vi "DataProcess.vi"(11 "Scan parameters":T1={"area/um"=36.9778, "range_x/v"=0.6347, "range_y/v"=0.7773, "interval/um"=0.1, "x_center/v"=3.35, "y_center/v"=5.55, "theta_1/de"=0.0, "theta_2/de"=60.0, "theta_3/de"=120.0}) -> (0 "ystart":dbl, 1 "xstart":dbl, 2 "ystep":dbl, 3 "xstep":dbl, 5 "NUM":i32)   [LabVIEW 2014]
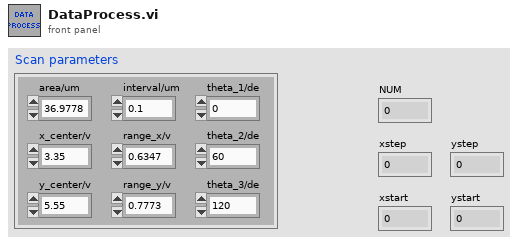
[diagram p1: front panel]
types:
  T1 = cluster{"area/um":dbl, "range_x/v":dbl, "range_y/v":dbl, "interval/um":dbl, "x_center/v":dbl, "y_center/v":dbl, "theta_1/de":dbl, "theta_2/de":dbl, "theta_3/de":dbl}
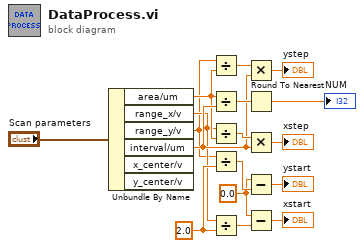
[diagram p0: block diagram]
diagram:
  w2 = 0.0 ("x")
  w9 = 2.0 ("y")
  n1 = Unbundle By Name("Scan parameters") -> ("area/um"=w12:dbl, "range_x/v"=w8:dbl, "range_y/v"=w7:dbl, "interval/um"=w13:dbl)  [unwired: 2 out]
  n2 = Divide(x=w7, y=w12) -> (x/y=w15:dbl)
  n3 = Divide(x=w12, y=w13) -> (x/y=w14:dbl)
  n4 = Divide(x=w8, y=w12) -> (x/y=w16:dbl)
  n5 = Divide(x=w7, y=w9) -> (x/y=w5:dbl)
  n6 = Divide(x=w8, y=w9) -> (x/y=w6:dbl)
  n7 = Multiply(x=w15, y=w13) -> (x*y=→"ystep":dbl)
  n8 = Round To Nearest(number=w14) -> (nearest integer value=→"NUM":dbl)
  n9 = Multiply(x=w16, y=w13) -> (x*y=→"xstep":dbl)
  n10 = Subtract(x=w2, y=w5) -> (x-y=→"ystart":dbl)
  n11 = Subtract(x=w2, y=w6) -> (x-y=→"xstart":dbl)
